vi "BK Precision 911X Series Create and Save Sequence.vi"() -> ()   [LabVIEW 2020]
doc: "This example demonstrates how to create a simple step sequence, store it into internal memory, and then run it."
uses:
  BK Precision 911X Series.lvlib
panel:
  in  "Active Steps (0000000000)":bool[](array[boolean])
  in  "Sequence Number (1)":dbl=1.0 min=1.0 max=10.0 step=1.0 format="%#.0p"
  in  "Step Slope":dbl[](array[numeric])=[1.0, 1.0, 1.0, 1.0, 1.0, 1.0, 1.0, 1.0, 1.0, 1.0] min=0.0010000000474974513 max=65.53500366210938 step=0.0010000000474974513 format="%.3f"
  in  "Step Width":dbl[](array[numeric])=[1.0, 1.0, 1.0, 1.0, 1.0, 1.0, 1.0, 1.0, 1.0, 1.0] min=0.001 max=65.535 step=0.001 format="%.3f"
  in  "Step Current":dbl[](array[numeric])=[1.0, 1.0, 1.0, 1.0, 1.0, 1.0, 1.0, 1.0, 1.0, 1.0] format="%.3g"
  in  "Step Voltage":dbl[](array[numeric])=[1.0, 1.0, 1.0, 1.0, 1.0, 1.0, 1.0, 1.0, 1.0, 1.0] format="%.3g"
  in  "VISA resource name":refnum<visa-resource-name>
  # "(c) 2013 B&K Precision Corporation.  ALL RIGHTS RESERVED."
  # "The instrument's list mode (sequence program) functionality is divided into two parts: Sequence (which contains all the step information), and List (which selects the sequences to run in the program).  Use this example to create the steps for the sequence first.  If any steps are not enabled from the Active Steps control, you can still input their corresponding Step Voltage, Current, Width, and Slope.  It will be stored into the instrument's internal memory, but will be skipped in the actual program if it's disabled.  Afterwards, configure the List using the Setup List Program.vi example to select the sequences you want to run."
  # "Steps   #  1   2    3   4    5   6   7    8   9   0"
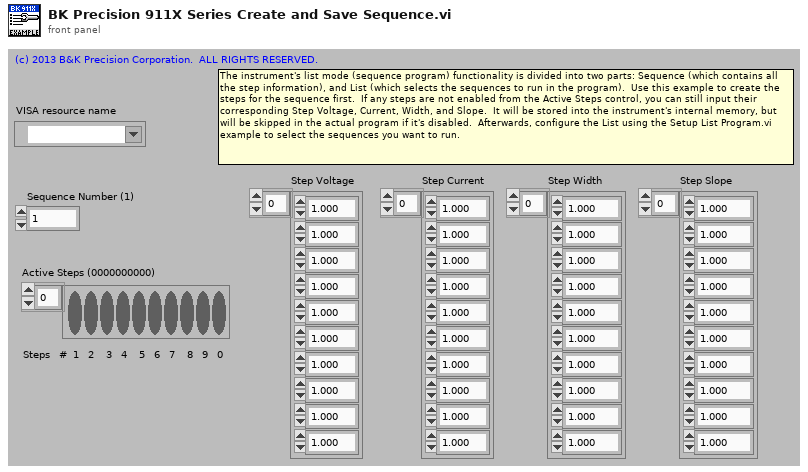
[diagram p1: front panel]
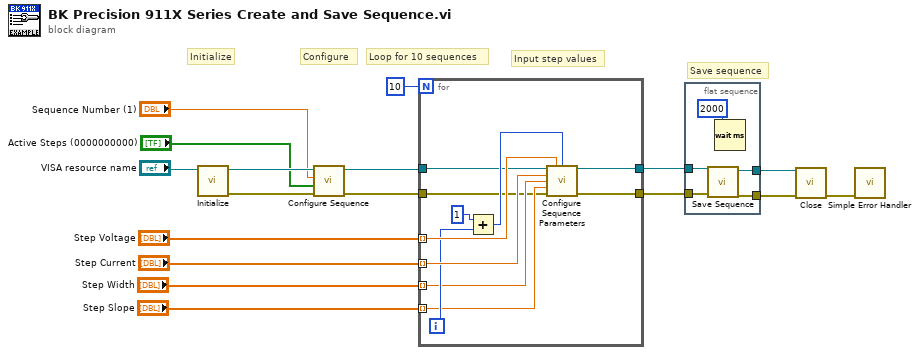
[diagram p0: block diagram]
diagram:
  # "Loop for 10 sequences"
  # "Input step values"
  # "Configure"
  # "Save sequence"
  # "Initialize"
  n1 = call "Initialize.vi"("VISA resource name"="VISA resource name") -> ("error out"=w14:errorcluster, "VISA resource name out"=w15:refnum<visa-resource-name>)  [unwired: 9 in]
  n2 = call "Configure Sequence.vi"("error in (no error)"=w14, "Active Steps (0000000000)"="Active Steps (0000000000)", "Sequence Number (1)"="Sequence Number (1)", "VISA resource name"=w15) -> ("error out"=w8:errorcluster, "VISA resource name out"=w2:refnum<visa-resource-name>)  [unwired: 6 in]
  n3 = for {
    N: 10 -> [_]
    tunnel: "Step Voltage" -> [w28] mode=indexing
    tunnel: "Step Current" -> [w27] mode=indexing
    tunnel: "Step Width" -> [w24] mode=indexing
    tunnel: "Step Slope" -> [w23] mode=indexing
    tunnel: w2 -> [w19]
    tunnel: [w20] -> w7
    tunnel: w8 -> [w21]
    tunnel: [w18] -> w1
    i -> [w26]
    n4 = Add(x=1, y=w26) -> (x+y=w22:i32)
    n5 = call "Configure Sequence Parameters.vi"("VISA resource name"=w19, "Step Voltage (1.000)"=w28, "Step Number (1)"=w22, "Step Current (1.000)"=w27, "Step Width (1)"=w24, "Step Slope (1)"=w23, "error in (no error)"=w21) -> ("VISA resource name out"=w20:refnum<visa-resource-name>, "error out"=w18:errorcluster)  [unwired: 7 in]
  }
  n6 = flat-sequence {
    tunnel: w7 -> [w32]
    tunnel: w1 -> [w31]
    tunnel: [w30] -> w6
    tunnel: [w29] -> w5
    frame #0 {
      n7 = call "Save Sequence.vi"("error in (no error)"=w31, "VISA resource name"=w32) -> ("error out"=w29:errorcluster, "VISA resource name out"=w30:refnum<visa-resource-name>)  [unwired: 8 in]
      n8 = Wait (ms)(milliseconds to wait=2000) -> ()  [unwired: 1 out]
    }
  }
  n9 = call "Close.vi"("error in (no error)"=w5, "VISA resource name"=w6) -> ("error out"=w16:errorcluster)  [unwired: 9 in]
  n10 = call <vilib>:"Simple Error Handler.vi"("error in (no error)"=w16) -> ()  [unwired: 4 in, 5 out]
